vi "Slave1.vi"() -> ()   [LabVIEW 2012]
uses:
  MyGlobals.vi
panel:
  out "Slave1Text":string
  in  "Slave1 Original":string="My "
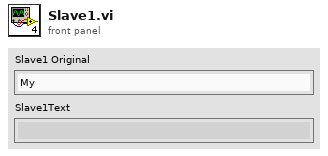
[diagram p1: front panel]
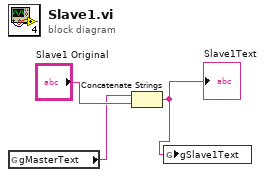
[diagram p0: block diagram]
diagram:
  n1 = global read "MyGlobals.vi" "gMasterText"() -> (w1:string)
  n2 = Concatenate Strings(w1, "Slave1 Original") -> (w3:string)
  "Slave1Text" <- w3
  n3 = global write "MyGlobals.vi" "gSlave1Text"(w3) -> ()
